vi "音訊分析.vi"() -> ()   [LabVIEW 2015]
uses:
  <vilib>/sound2/lvsound2.llb/Sampling Mode.ctl
  <vilib>/sound2/lvsound2.llb/Sound Data Format.ctl
  <vilib>/Analysis/1siggen.llb/Ramp Pattern by Samples.vi
  <vilib>/Analysis/2dsp.llb/Real FFT.vi
  <vilib>/sound2/lvsound2.llb/Sound Input Read (DBL).vi
  <vilib>/Analysis/NI_AALPro.lvlib
  <vilib>/Analysis/NI_AALBase.lvlib
panel:
  out "element":dbl
  out "Ramp Pattern 2":dbl[](array[numeric])
  out "Ramp Pattern":dbl[](array[numeric])
  out "XY Graph":cluster{dbl[], "Ramp Pattern":dbl[]}(graph)
  in  "stop":bool
  out "Waveform Graph":waveform(dbl)[](graph)
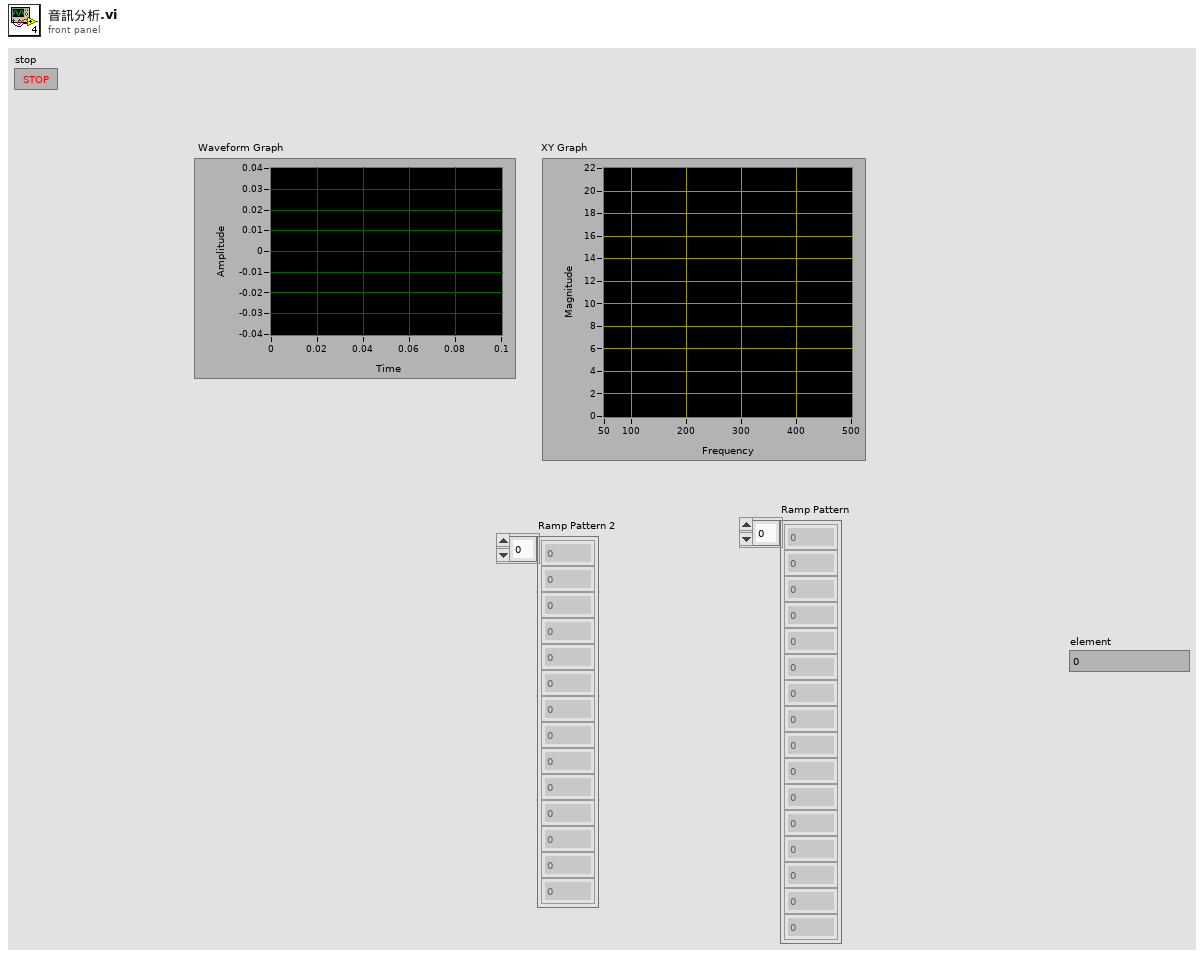
[diagram p1: front panel]
types:
  T1 = typedef "Sound Data Format.ctl" = cluster{"sample rate (S/s)":dbl, "number of channels":i32, "bits per sample":i32}
  T2 = typedef "Sampling Mode.ctl" = i32
  T3 = typedef "Sound Input Task ID.ctl" = u32
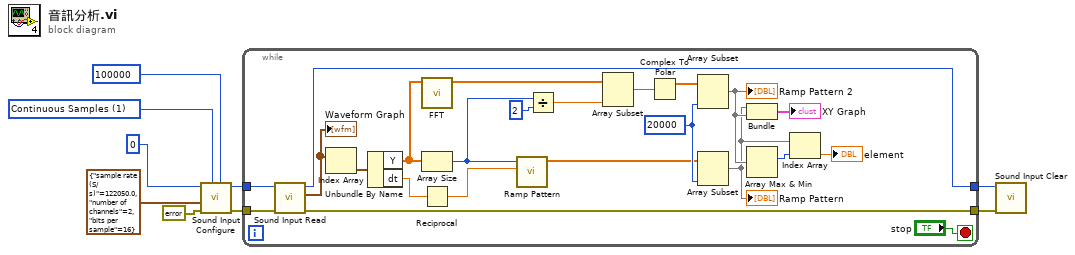
[diagram p0: block diagram]
diagram:
  w4 = T2 1 items=["Finite Samples", "Continuous Samples"] ("sample mode")
  n1 = call <vilib>:"Sound Input Configure.vi"("number of samples/ch"=100000, "sample mode"=w4, "error in (no error)"=errorcluster {"status"=FALSE, "code"=0, "source"=""}, "sound format"=T1 {"sample rate (S/s)"=122050.0, "number of channels"=2, "bits per sample"=16}, "device ID"=u32 0) -> ("error out"=w6:errorcluster, "task ID"=w9:T3)  [unwired: 5 in]
  n2 = while {
    tunnel: w9 -> [w32]
    tunnel: [w31] -> w8
    tunnel: [w30] -> w7
    tunnel: w6 -> [w29]
    stop <- "stop" stop-if-true
    w14 = 20000 ("length")
    n3 = call-poly <vilib>:"Sound Input Read.vi"("error in (no error)"=w29, "task ID"=w32) -> ("error out"=w30:errorcluster, "data"=w27:waveform(dbl)[], "task ID out"=w31:T3)  [unwired: 7 in]
    "Waveform Graph" <- w27
    n4 = Index Array(array=w27) -> (element=w26:waveform(dbl))  [unwired: 1 in]
    n5 = Unbundle By Name(w26) -> ("Y"=w25:dbl[], "dt"=w20:dbl)
    n6 = call-poly <vilib>:"FFT.vi"("X"=w25) -> ("FFT {X}"=w23:cdb[])  [unwired: 9 in, 1 out]
    n7 = Array Size(array=w25) -> (size(s)=w18:i32)
    n8 = Reciprocal(x=w20) -> (1/x=w19:dbl)
    n9 = call-poly <vilib>:"Ramp Pattern.vi"("end"=w19, "samples"=w18) -> ("Ramp Pattern"=w11:dbl[])  [unwired: 8 in, 1 out]
    n10 = Divide(x=w18, y=2) -> (x/y=w22:dbl)
    n11 = Array Subset(array=w23, length=w22) -> (w21:cdb[])  [unwired: 1 in]
    n12 = Complex To Polar(r * e^(i*theta)=w21) -> (r=w13:dbl[])  [unwired: 1 out]
    n13 = Array Subset(array=w13, length=w14) -> (w12:dbl[])  [unwired: 1 in]
    "Ramp Pattern 2" <- w12
    n14 = Array Subset(array=w11, length=w14) -> (w10:dbl[])  [unwired: 1 in]
    "Ramp Pattern" <- w10
    n15 = Bundle(w10, w12) -> (→"XY Graph":cluster{dbl[], dbl[]})  [unwired: 1 in]
    n16 = Array Max & Min(array=w12) -> (max index (indices)=w16:i32)  [unwired: 3 out]
    n17 = Index Array(array=w10, index=w16) -> (element=→"element":dbl)
  }
  n18 = call <vilib>:"Sound Input Clear.vi"("error in (no error)"=w7, "task ID"=w8) -> ()  [unwired: 9 in, 1 out]
